vi "Set_CHROMA.vi"(3 "instrument handle out":refnum<k15>) -> (11 "instrument handle":refnum<k15>)   [LabVIEW 2013]
uses:
  FT_HMI.llb/GLOBAL_PUMPS_PARAMS.vi
  FT_HMI.llb/GLOBAL_GEN.vi
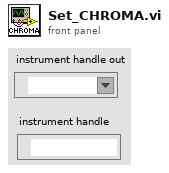
[diagram p1: front panel]
types:
  T1 = cluster{"VAC":cluster{"ENABLE":bool, "PUMPING_TIME [ms]":dbl, "MEASUREMENT_TIME [ms]":dbl, "PRESSURE_LIMIT [bar]":sgl}, "Q1":cluster{"ENABLE":bool, "PUMPING_TIME  [ms]":dbl, "MEASUREMENT_TIME  [ms]":sgl, "FLOW_TARGET  [ml/min]":sgl, "FLOW_LIMIT_UP  [ml/min]":sgl, "FLOW_LIMIT_DOWN [ml/min]":sgl, "PRESSURE_TARGET [bar]":sgl, "PRESSURE_LIMIT_UP [bar]":sgl, "PRESSURE_LIMIT_DOWN [bar]":sgl, "MAX_FLOW":bool}, "Q2":cluster{"ENABLE":bool, "PUMPING_TIME [ms]":dbl, "MEASUREMENT_TIME [ms]":dbl, "FLOW_TARGET [ml/min]":sgl, "FLOW_LIMIT_UP [ml/min]":sgl, "FLOW_LIMIT_DOWN [ml/min]":sgl, "PRESSURE_TARGET [bar]":sgl, "PRESSURE_LIMIT_UP [bar]":sgl, "PRESSURE_LIMIT_DOWN [bar]":sgl, "MAX_FLOW":bool}, "PMAX":cluster{"ENABLE":bool, "PUMPING_TIME [ms]":dbl, "MEASUREMENT_TIME [ms]":dbl, "PRESSURE_LIMIT [bar]":sgl, "PRESSURE_LOOSE_TIME [ms]":sgl}, "PRINT":cluster{"ENABLE":bool}, "SUPPLY":cluster{"VOLTAGE [V]":dbl, "FREQUENCY [Hz]":dbl}}
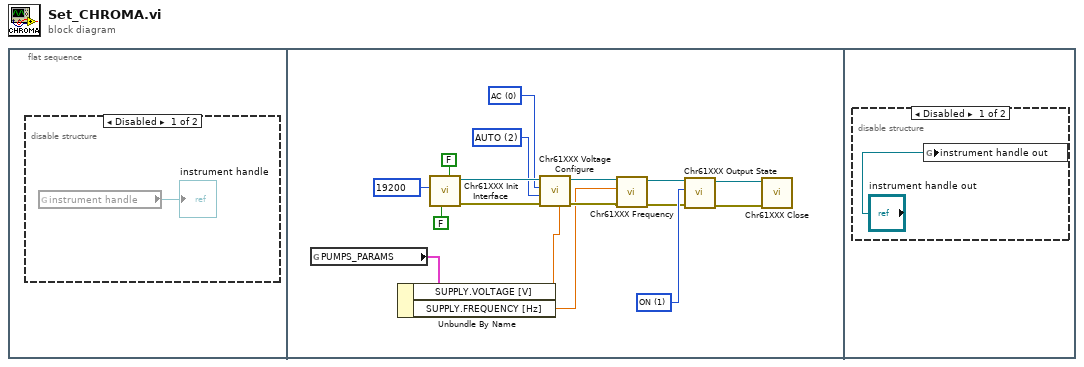
[diagram p0: block diagram]
diagram:
  n1 = flat-sequence {
    frame #0 {
      n2 = disable-structure shown="Disabled" {
        frame Disabled {
          n3 = global read "GLOBAL_GEN.vi" "instrument handle"() -> (→"instrument handle":refnum<k15>)
        }
        frame Enabled {
        }
      }
    }
    frame #1 {
      w7 = 19200 items=["9600"=9600, "19200"=19200, "38400"=38400, "57600"=57600, "115200"=115200] ("baud rate")
      w14 = 2 items=["LOW", "HIGH", "AUTO"] ("voltage range")
      w13 = 0 items=["AC", "DC"] ("voltage type")
      w10 = u16 1 items=["OFF", "ON"] ("state")
      n4 = global read "GLOBAL_PUMPS_PARAMS.vi" "PUMPS_PARAMS"() -> (w4:T1)
      n5 = Unbundle By Name(w4) -> ("SUPPLY.VOLTAGE [V]"=w3:dbl, "SUPPLY.FREQUENCY [Hz]"=w2:dbl)
      n6 = call <instrlib>:"Chr61XXX Init Interface.vi"("id query"=FALSE, "reset device"=FALSE, "baud rate"=w7) -> ("error out"=w15:errorcluster, "instrument handle out"=w16:refnum<k15>)  [unwired: 6 in, 1 out]
      n7 = call <instrlib>:"Chr61XXX Voltage Configure.vi"("voltage"=w3, "error in (no error)"=w15, "voltage range"=w14, "voltage type"=w13, "instrument handle"=w16) -> ("error out"=w9:errorcluster, "instrument handle out"=w12:refnum<k15>)  [unwired: 5 in]
      n8 = call <instrlib>:"Chr61XXX Frequency.vi"("error in (no error)"=w9, "frequency"=w2, "instrument handle"=w12) -> ("error out"=w8:errorcluster, "instrument handle out"=w11:refnum<k15>)  [unwired: 7 in]
      n9 = call <instrlib>:"Chr61XXX Output State.vi"("error in (no error)"=w8, "state"=w10, "instrument handle"=w11) -> ("error out"=w17:errorcluster, "instrument handle out"=w18:refnum<k15>)  [unwired: 7 in]
      n10 = call <instrlib>:"Chr61XXX Close.vi"("error in (no error)"=w17, "instrument handle"=w18) -> ()  [unwired: 9 in, 1 out]
    }
    frame #2 {
      n11 = disable-structure shown="Disabled" {
        frame Disabled {
          n12 = global write "GLOBAL_GEN.vi" "instrument handle out"("instrument handle out") -> ()
        }
        frame Enabled {
        }
      }
    }
  }
